vi "Timed interval image pair.vi"(0 "Image name":string="test", 1 "Image directory path":path=path "C:/test", 2 "Image pair interval (Sec)":dbl=0.1, 3 "Interface name":T1="cam0", 4 "VideoMode":u32=12) -> (5 "Measured interval (s)":dbl=6.776, 6 "Image acq. error(s)":errorcluster)   [LabVIEW 2014]
uses:
  <vilib>/userdefined/High Color/IMAQdx.ctl
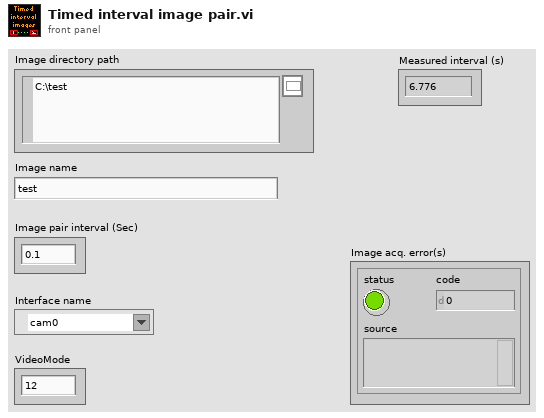
[diagram p1: front panel]
types:
  T1 = typedef "IMAQdx.ctl" = refnum<k21>
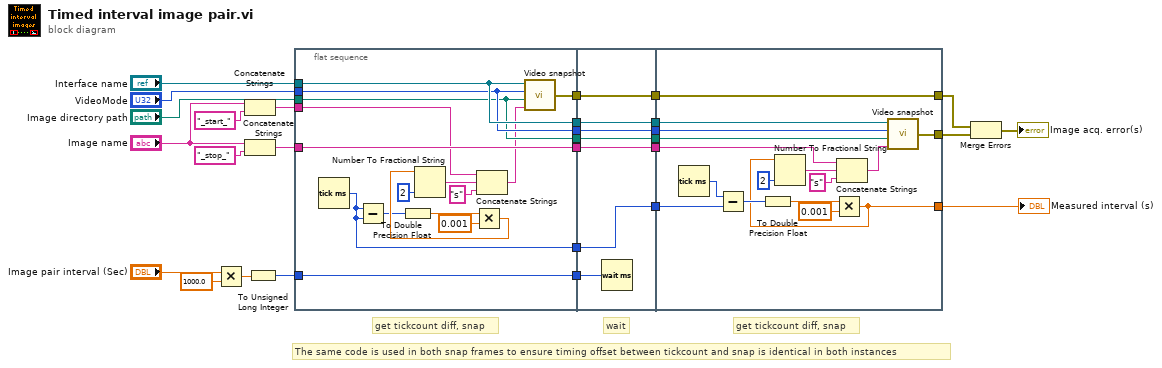
[diagram p0: block diagram]
diagram:
  # "The same code is used in both snap frames to ensure timing offset between tickcount and snap is identical in both instances"
  # "get tickcount diff, snap"
  # "wait"
  # "get tickcount diff, snap"
  n1 = Multiply(x="Image pair interval (Sec)", y=1000.0) -> (x*y=w29:dbl)
  n2 = Concatenate Strings("Image name", "_start_" ("string")) -> (w7:string)
  n3 = Concatenate Strings("Image name", "_stop_" ("string")) -> (w3:string)
  n4 = To Unsigned Long Integer(number=w29) -> (unsigned 32bit integer=w27:u32)
  n5 = flat-sequence {
    tunnel: w27 -> [w45]
    tunnel: [w45] -> w25
    tunnel: [w32] -> w23
    tunnel: [w44] -> w21
    tunnel: "Interface name" -> [w43]
    tunnel: [w43] -> w15
    tunnel: "VideoMode" -> [w42]
    tunnel: "Image directory path" -> [w41]
    tunnel: [w42] -> w11
    tunnel: [w41] -> w9
    tunnel: w7 -> [w34]
    tunnel: w3 -> [w40]
    tunnel: [w40] -> w1
    tunnel: w25 -> [w52]
    tunnel: [w51] -> w24
    tunnel: w23 -> [w51]
    tunnel: [w50] -> w22
    tunnel: w21 -> [w50]
    tunnel: [w49] -> w16
    tunnel: w15 -> [w49]
    tunnel: [w48] -> w12
    tunnel: w11 -> [w48]
    tunnel: [w47] -> w10
    tunnel: w9 -> [w47]
    tunnel: [w46] -> w2
    tunnel: w1 -> [w46]
    tunnel: w24 -> [w67]
    tunnel: w22 -> [w65]
    tunnel: [w66] -> w19
    tunnel: [w65] -> w20
    tunnel: w16 -> [w64]
    tunnel: w12 -> [w63]
    tunnel: w10 -> [w62]
    tunnel: [w53] -> w4
    tunnel: w2 -> [w57]
    frame #0 {
      n6 = Tick Count (ms)() -> (millisecond timer value=w32:u32)
      n7 = Subtract(x=w32, y=w32) -> (x-y=w37:u32)
      n8 = To Double Precision Float(number=w37) -> (double precision float=w36:dbl)
      n9 = Multiply(x=w36, y=0.001) -> (x*y=w39:dbl)
      n10 = Number To Fractional String(number=w39, precision (6)=i16 2) -> (F-format string=w30:string)  [unwired: 2 in]
      n11 = Concatenate Strings(w34, w30, "s" ("string")) -> (w33:string)
      n12 = call "Video snapshot.vi"("Image name"=w33, "Image directory path"=w41, "VideoMode"=w42, "Interface name"=w43) -> ("Error Out"=w44:errorcluster)
    }
    frame #1 {
      n13 = Wait (ms)(milliseconds to wait=w52) -> ()  [unwired: 1 out]
    }
    frame #2 {
      n14 = Tick Count (ms)() -> (millisecond timer value=w68:u32)
      n15 = Subtract(x=w68, y=w67) -> (x-y=w59:u32)
      n16 = To Double Precision Float(number=w59) -> (double precision float=w60:dbl)
      n17 = Multiply(x=w60, y=0.001) -> (x*y=w53:dbl)
      n18 = Number To Fractional String(number=w53, precision (6)=i16 2) -> (F-format string=w56:string)  [unwired: 2 in]
      n19 = Concatenate Strings(w57, w56, "s" ("string")) -> (w54:string)
      n20 = call "Video snapshot.vi"("Image name"=w54, "Image directory path"=w62, "VideoMode"=w63, "Interface name"=w64) -> ("Error Out"=w66:errorcluster)
    }
  }
  n21 = Merge Errors(w20, w19) -> (→"Image acq. error(s)":errorcluster)
  "Measured interval (s)" <- w4
